vi "Change Inheritance.vi"(8 "error in (no error)":errorcluster, 10 "Parent Class":refnum<vi>, 11 "LV Class Ref in":refnum<vi>) -> (0 "error out":errorcluster, 3 "LV Class ref out":refnum<vi>)   [LabVIEW 2019, in "gRPC Template Creation Utility.lvlib"]
uses:
  gRPC Template Creation Utility.lvlib
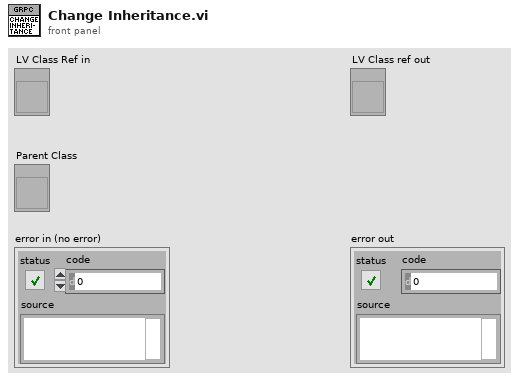
[diagram p1: front panel]
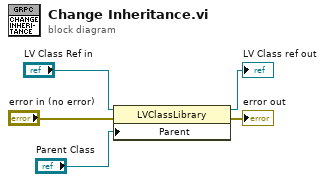
[diagram p0: block diagram]
diagram:
  n1 = property class="LVClassLibrary"(reference="LV Class Ref in", error in="error in (no error)", "Parent"="Parent Class") -> (reference out=→"LV Class ref out":refnum<vi>, error out=→"error out":errorcluster)
